vi "Position Control.vi"(8 "error in (no error)":errorcluster, 11 "Control Panel in":refnum<class "Control Panel.lvclass">) -> (0 "error out":errorcluster, 3 "Control Panel out":refnum<class "Control Panel.lvclass">)   [LabVIEW 2019, in "Control Panel.lvlib" / "Control Panel.lvclass"]
uses:
  Control Panel.lvclass
  <vilib>/Rock Robotics/WPI/ThirdParty/Phoenix-LabVIEW/Motor Controller/Controls/CTRE_Phoenix_MotorControl_ControlMode.ctl
panel:
  out "Matched Color":cluster{"R":dbl, "G":dbl, "B":dbl}
  out "Matched Color Name":string
  out "Turns to get to target":dbl
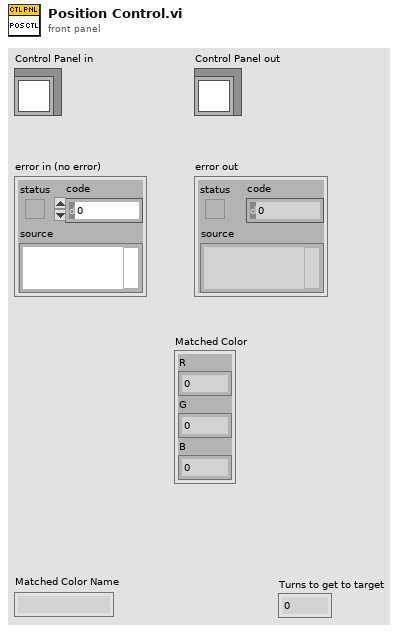
[diagram p1: front panel]
types:
  T1 = typedef "CTRE_Phoenix_MotorControl_ControlMode.ctl" = u16
  T2 = typedef "Color Sensor V3 DevRef.ctl" = cluster{"I2CDevRef":T3}
  T3 = typedef "WPI_I2CDevRef.ctl" = cluster{"DevStatus":errorcluster, "Device Address":u8, "Handle":i32, "I2C Bus":T4}
  T4 = typedef "i2c_bus.ctl" = enum16{"I2C On-Board", "I2C MXP", "Invalid"}
  T5 = typedef "WPI_MotorControlDeviceRef.ctl" = cluster{"DeviceStatus":errorcluster, "Type":T6, "PWM":cluster{"PWM Channel":T7, "DeadBand":T8}, "CAN":cluster{"Device Number":u8, "SetOutput VI Ref":variant, "GetOutput VI Ref":variant, "Enable VI Ref":variant, "Disable VI Ref":variant, "Data":variant}, "Invert":bool, "DIO PWM":cluster{"PWM \"Enable\" Channel":T7, "DIOChannel":T9, "PWM Rate":dbl}}
  T6 = typedef "WPI_MotorControlType.ctl" = enum16{"PWM", "CAN", "DIO PWM"}
  T7 = typedef "FPGA_DIOPWMChannel.ctl" = enum8{"PWM 0", "PWM 1", "PWM 2", "PWM 3", "PWM 4", "PWM 5", "PWM 6", "PWM 7", "PWM 8", "PWM 9", "PWM MXP 0", "PWM MXP 1", "PWM MXP 2", "PWM MXP 3", "PWM MXP 4", "PWM MXP 5", "PWM MXP 6", "PWM MXP 7", "PWM MXP 8", "PWM MXP 9", "Invalid"}
  T8 = typedef "WPI_PWMDeadband.ctl" = cluster{"Name":string, "maxPositivePwm":i32, "minPositivePwm":i32, "centerPwm":i32, "maxNegativePwm":i32, "minNegativePwm":i32, "angularRange":u16}
  T9 = typedef "FPGA_DIOChannel.ctl" = enum8{"DIO 0", "DIO 1", "DIO 2", "DIO 3", "DIO 4", "DIO 5", "DIO 6", "DIO 7", "DIO 8", "DIO 9", "DIO MXP 0", "DIO MXP 1", "DIO MXP 2", "DIO MXP 3", "DIO MXP 4", "DIO MXP 5", "DIO MXP 6", "DIO MXP 7", "DIO MXP 8", "DIO MXP 9", "DIO MXP 10", "DIO MXP 11", "DIO MXP 12", "DIO MXP 13", "DIO MXP 14", "DIO MXP 15", "SPI Port CS1", "SPI Port CS2", "SPI Port CS3", "SPI Port MISO", "SPI Port MOSI", "Invalid"}
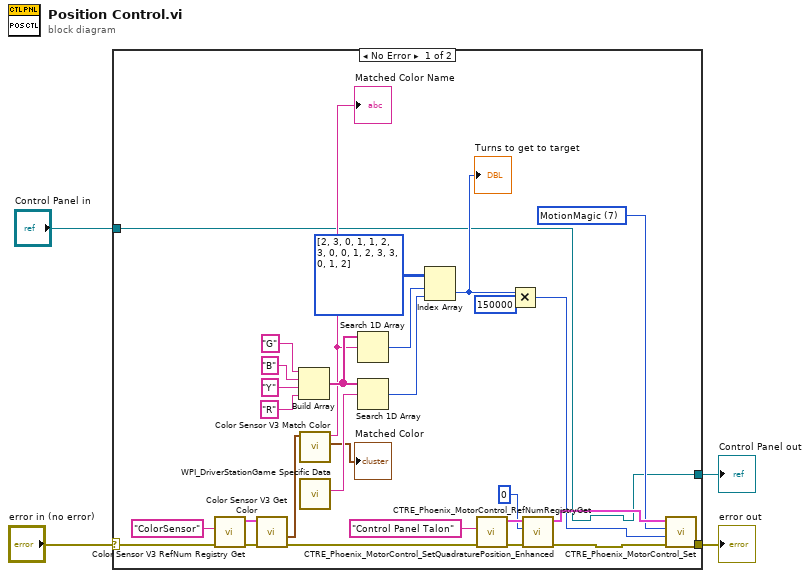
[diagram p0: block diagram]
diagram:
  n1 = case shown="No Error" "error in (no error)" {
    selector: "error in (no error)" -> [w16 w35]
    tunnel: [w8 w35] -> w3
    tunnel: [w6 w34] -> w1
    tunnel: "Control Panel in" -> [w6 w34]
    frame No Error {
      w9 = T1 7 items=["PercentOutput"=0, "Position"=1, "Velocity"=2, "Current"=3, "Follower"=5, "MotionProfile"=6, "MotionMagic"=7, "MotionProfileArc"=10, "Disabled"=15] ("Control Mode")
      n2 = call <vilib>:"Color Sensor V3 RefNum Registry Get.vi"("error in (no error)"=w16, "refnum name"="ColorSensor") -> ("error out"=w27:errorcluster, "ColorSensorDevRef"=w26:T2)  [unwired: 8 in]
      n3 = call <vilib>:"Color Sensor V3 Get Color.vi"("error in (no error)"=w27, "ColorSensorDevRef"=w26) -> ("error out"=w15:errorcluster, "Normalized Color"=w28:cluster{"R":dbl, "G":dbl, "B":dbl})  [unwired: 6 in, 2 out]
      n4 = Build Array("G", "B", "Y", "R") -> (w29:string[])
      n5 = call <vilib>:"Color Sensor V3 Match Color.vi"("Measured Color"=w28) -> ("Matched Color"=→"Matched Color":cluster{"R":dbl, "G":dbl, "B":dbl}, "Matched Color Name"=w18:string)  [unwired: 8 in, 1 out]
      "Matched Color Name" <- w18
      n6 = call <vilib>:"WPI_DriverStationGame Specific Data.vi"() -> ("Game Specific Data"=w33:string)  [unwired: 11 in]
      n7 = Search 1D Array(1D array=w29, element=w18) -> (index of element=w31:i32)  [unwired: 1 in]
      n8 = Search 1D Array(1D array=w29, element=w33) -> (index of element=w30:i32)  [unwired: 1 in]
      n9 = Index Array(array=i32[][] [[2, 3, 0, 1], [1, 2, 3, 0], [0, 1, 2, 3], [3, 0, 1, 2]], index (row)=w31, index (col)=w30) -> (element=w32:i32)
      "Turns to get to target" <- w32
      n10 = call <vilib>:"CTRE_Phoenix_MotorControl_RefNumRegistryGet.vi"("error in (no error)"=w15, "refnum name"="Control Panel Talon") -> ("error out"=w14:errorcluster, "PhoenixMotorControlDevRef"=w13:T5)  [unwired: 8 in]
      n11 = Multiply(x=w32, y=150000) -> (x*y=w5:i32)
      n12 = call <vilib>:"CTRE_Phoenix_MotorControl_SetQuadraturePosition_Enhanced.vi"("error in (no error)"=w14, "New Position"=0, "PhoenixMotorControlDevRef"=w13) -> ("error out"=w7:errorcluster, "PhoenixMotorControlDevRef"=w10:T5)  [unwired: 7 in]
      n13 = call <vilib>:"CTRE_Phoenix_MotorControl_Set.vi"("error in (no error)"=w7, "Output"=w5, "Control Mode"=w9, "PhoenixMotorControlDevRef"=w10) -> ("error out"=w8:errorcluster)  [unwired: 6 in, 1 out]
    }
    frame Error {
    }
  }
  "error out" <- w3
  "Control Panel out" <- w1
